vi "fgv_erp42-232.vi"(7 "cmd":enum16{"init", "read", "write", "close"}(ring), 8 "error in":errorcluster) -> (0 "error out":errorcluster, 2 "valid":bool, 3 "read_buffer":string)   [LabVIEW 2019]
uses:
  <vilib>/Instr/_visa.llb/VISA Configure Serial Port (Instr).vi
panel:
  out "send_data":u8[](array[numeric]) format="%x"
  out "ERP_Receive":T1
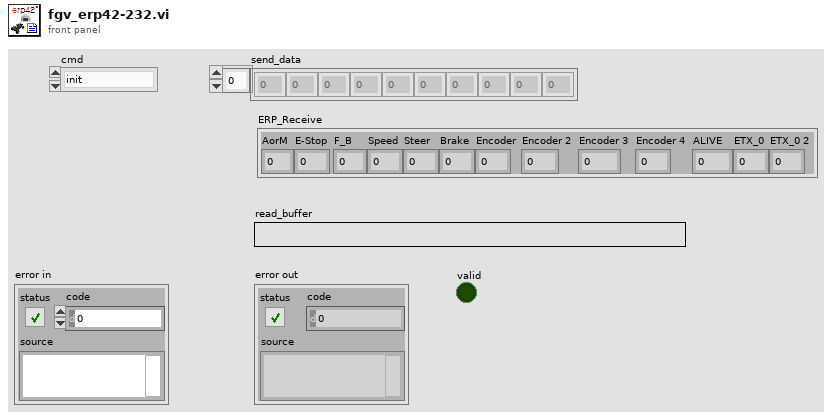
[diagram p1: front panel]
types:
  T1 = cluster{"AorM":u8, "E-Stop":u8, "F_B":u8, "Speed":u16, "Steer":i16, "Brake":u8, "Encoder":u8, "Encoder 2":u8, "Encoder 3":u8, "Encoder 4":u8, "ALIVE":u8, "ETX_0":u8, "ETX_0 2":u8}
  T2 = cluster{"Port":refnum<visa-resource-name>, "speed limits":cluster{"speed-limit":dbl, "steer-limit":dbl}, "limits":cluster{"speed limits":cluster{"max":dbl, "min":dbl}, "steer limits":cluster{"max":dbl, "min":dbl}}}
  T3 = cluster{"Dir":u8, "Acc_set":u16, "Steer_set":i16, "Brake":i16, "Direction":bool, "speed_curr":dbl, "steer_curr":i16, "brake_curr":i16, "Acc_now":i16}
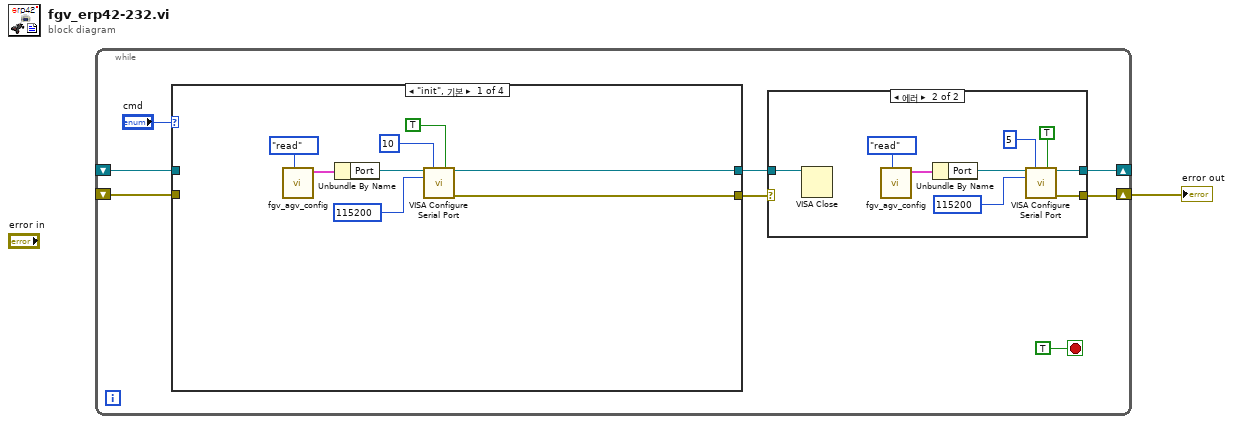
[diagram p0: block diagram]
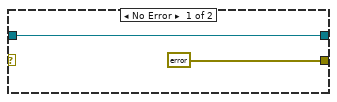
[diagram p2: hidden frame]
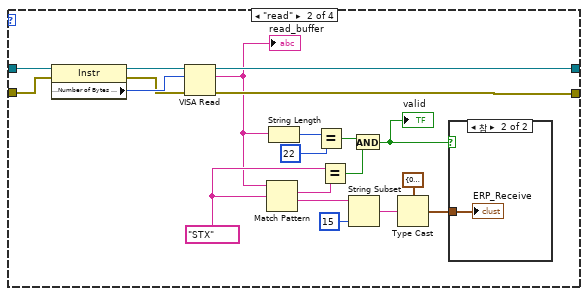
[diagram p3: hidden frame]
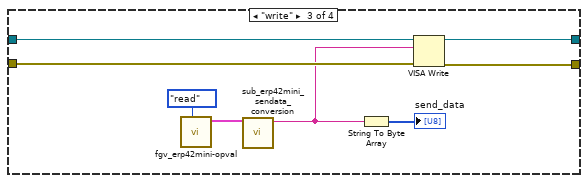
[diagram p5: hidden frame]
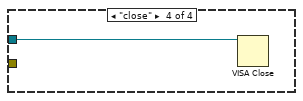
[diagram p6: hidden frame]
diagram:
  n1 = while {
    shift-right: [w4] -> _
    shift-left: _ -> [w7]
    shift-right: [w3] -> w1
    shift-left: _ -> [w6]
    stop <- TRUE stop-if-true
    n2 = case shown="\"init\", 기본" "cmd" {
      tunnel: [w28 w45 w55 _] -> w5
      tunnel: [w26 w44 w54 _] -> w2
      tunnel: w7 -> [_ w48 w56 w58]
      tunnel: w6 -> [_ w42 w57 _]
      frame "init", Default {
        n3 = call "fgv_agv_config.vi"("cmd"=enum16{"read", "write"}."read") -> ("AGV cfg out"=w23:T2)  [unwired: 9 in, 1 out]
        n4 = Unbundle By Name(w23) -> ("Port"=w22:refnum<visa-resource-name>)
        n5 = call-poly "VISA Configure Serial Port"("VISA resource name"=w22, "timeout (10sec)"=u32 10, "Enable Termination\nChar (T)"=TRUE ("Enable Termination\nChar (T)"), "baud rate (9600)"=u32 115200) -> ("VISA resource name out"=w28:refnum<visa-resource-name>, "error out"=w26:errorcluster)  [unwired: 10 in]
      }
      frame "read" {
        w36 = "STX" ("검색 문자열/문자 (-)")
        n6 = property class="Instr"(reference=w48, error in=w42) -> (reference out=w46:refnum<visa-resource-name>, error out=w43:errorcluster, "Serial Settings:Number of Bytes at Serial Port"=w47:u32)
        n7 = VISA Read(VISA resource name=w46, byte count=w47, error in (no error)=w43) -> (VISA resource name out=w45:refnum<visa-resource-name>, read buffer=w34:string, error out=w44:errorcluster)  [unwired: 1 out]
        "read_buffer" <- w34
        n8 = Match Pattern(string=w34, regular expression=w36) -> (match substring=w39:string, after substring=w38:string)  [unwired: 1 in, 2 out]
        n9 = String Length(string=w34) -> (length=w33:i32)
        n10 = Equal?(x=w33, y=22 ("Numeric")) -> (x = y?=w29:bool)
        n11 = Equal?(x=w36, y=w39) -> (x = y?=w30:bool)
        n12 = String Subset(string=w38, length (rest)=15 ("길이(나머지)")) -> (substring=w40:string)  [unwired: 1 in]
        n13 = And(x=w29, y=w30) -> (x .and. y?=w31:bool)
        "valid" <- w31
        n14 = Type Cast(type=T1 {"AorM"=0, "E-Stop"=0, "F_B"=0, "Speed"=0, "Steer"=0, "Brake"=0, "Encoder"=0, "Encoder 2"=0, "Encoder 3"=0, "Encoder 4"=0, "ALIVE"=0, "ETX_0"=13, "ETX_0 2"=10}, x=w40) -> (*(type *) &x=w41:T1)
        n15 = case shown="참" w31 {
          tunnel: w41 -> [_ w49]
          frame False {
          }
          frame True {
            "ERP_Receive" <- w49
          }
        }
      }
      frame "write" {
        n16 = call "fgv_erp42mini-opval.vi"("cmd"=enum16{"ini", "read", "wirte"}."read") -> ("car_v_out"=w51:T3)  [unwired: 10 in]
        n17 = call "sub_erp42mini_sendata_conversion.vi"("car_v"=w51) -> ("drive_v_strout"=w52:string)  [unwired: 10 in]
        n18 = String To Byte Array(string=w52) -> (unsigned byte array=→"send_data":u8[])
        n19 = VISA Write(VISA resource name=w56, write buffer=w52, error in (no error)=w57) -> (VISA resource name out=w55:refnum<visa-resource-name>, error out=w54:errorcluster)  [unwired: 1 out]
      }
      frame "close" {
        n20 = VISA Close(VISA resource name=w58) -> ()  [unwired: 1 in, 1 out]
      }
    }
    n21 = case shown="에러" w2 {
      tunnel: w5 -> [w11 w20]
      tunnel: [w11 w17] -> w4
      tunnel: [errorcluster {"status"=FALSE, "code"=0, "source"=""} ("error out") w16] -> w3
      frame No Error {
      }
      frame Error {
        n22 = VISA Close(VISA resource name=w20) -> ()  [unwired: 1 in, 1 out]
        n23 = call "fgv_agv_config.vi"("cmd"=enum16{"read", "write"}."read") -> ("AGV cfg out"=w14:T2)  [unwired: 9 in, 1 out]
        n24 = Unbundle By Name(w14) -> ("Port"=w13:refnum<visa-resource-name>)
        n25 = call-poly "VISA Configure Serial Port"("VISA resource name"=w13, "timeout (10sec)"=u32 5, "Enable Termination\nChar (T)"=TRUE ("Enable Termination\nChar (T)"), "baud rate (9600)"=u32 115200) -> ("VISA resource name out"=w17:refnum<visa-resource-name>, "error out"=w16:errorcluster)  [unwired: 10 in]
      }
    }
  }
  "error out" <- w1
